vi "Get Absolute Source Dir Path.vi"() -> (0 "error out":errorcluster, 3 "source dir":path)   [LabVIEW 2021]
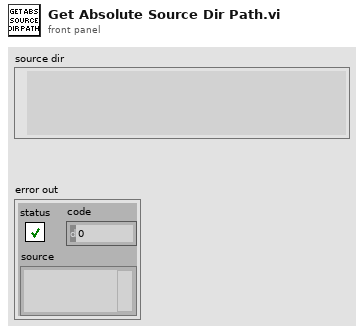
[diagram p1: front panel]
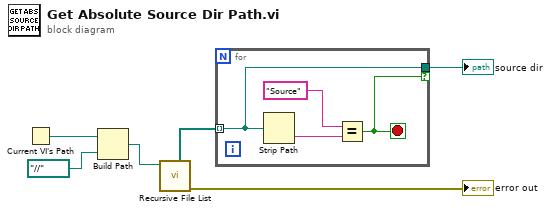
[diagram p0: block diagram]
diagram:
  n1 = Current VI's Path() -> (path=w6:path)
  n2 = Build Path(base path=w6, name or relative path=path "../../..") -> (appended path=w4:path)
  n3 = call <vilib>:"Recursive File List.vi"("Folder Path"=w4) -> ("error out"=→"error out":errorcluster, "All Folders"=w3:path[])  [unwired: 6 in, 3 out]
  n4 = for {
    tunnel: w3 -> [w8] mode=indexing
    tunnel: [w8] -> w1 if=w7
    stop <- w7 stop-if-true
    n5 = Strip Path(path=w8) -> (name=w10:string)  [unwired: 1 out]
    n6 = Equal?(x="Source", y=w10) -> (x = y?=w7:bool)
  }
  "source dir" <- w1
